vi "CAL_FLOW_SENSOR 2016.vi"(7 "Array in":refnum<k24>[](array[refnum]), 8 "error in (no error)":errorcluster, 9 "Descriptions":string[](array[string]), 11 "flow_slope_IN":dbl=51.35 format="%.2f") -> (0 "error out":errorcluster, 2 "Sensor Cluster":T1, 3 "flow_slope\nmL/min":dbl=51.35 format="%.2f", 5 "Array out":refnum<k24>[](array[refnum]))   [LabVIEW 2016]
uses:
  C:/Program Files (x86)/National Instruments/LabVIEW 2016/vi.lib/ULx/ULx_LV.dll
  Program Files (x86)/National Instruments/LabVIEW 2016/vi.lib/ULx/ULx_LV.dll
  controls/MCC DAQ Readings.ctl
  Kpro Globals.vi
  Global_SIM_switch.vi
panel:
  out "Global Flow\n Slope Valid":bool
  in  "Flow Slope":dbl format="%#_13g"
  out "Flow":dbl format="%.2f"
  in  "stop":bool
  in  "start":bool
  # "FLOW SENSOR CALIBRATION"
  # "Start Kpro flow. Allow the flow to equilibrate."
  # "After flow has equilibrated,  Press Start, simultaneously move Kpro effluent into graduated cylinder."
  # "Press Stop when 100 mL of water has been collected."
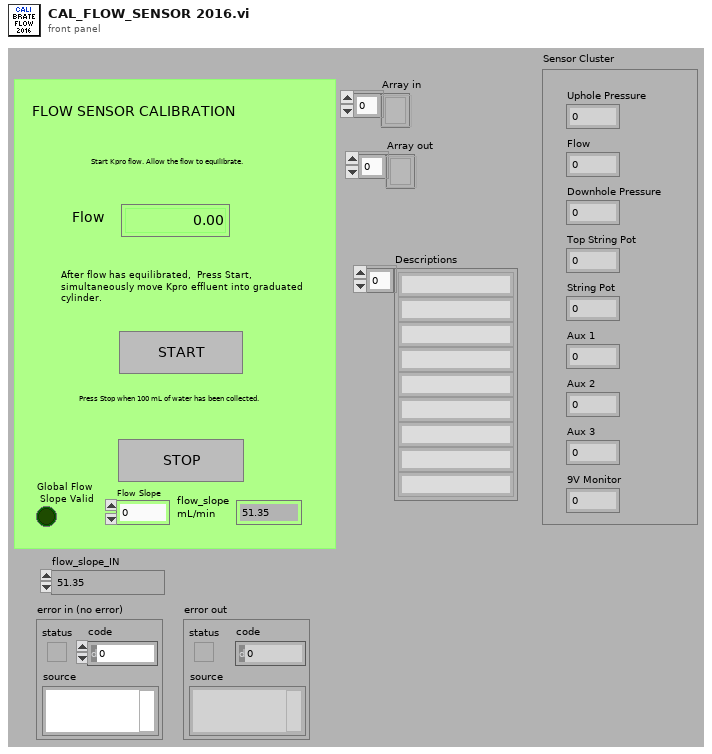
[diagram p1: front panel]
types:
  T1 = typedef "MCC DAQ Readings.ctl" = cluster{"Uphole Pressure":dbl, "Flow":dbl, "Downhole Pressure":dbl, "Top String Pot":dbl, "String Pot":dbl, "Aux 1":dbl, "Aux 2":dbl, "Aux 3":dbl, "9V Monitor":dbl}
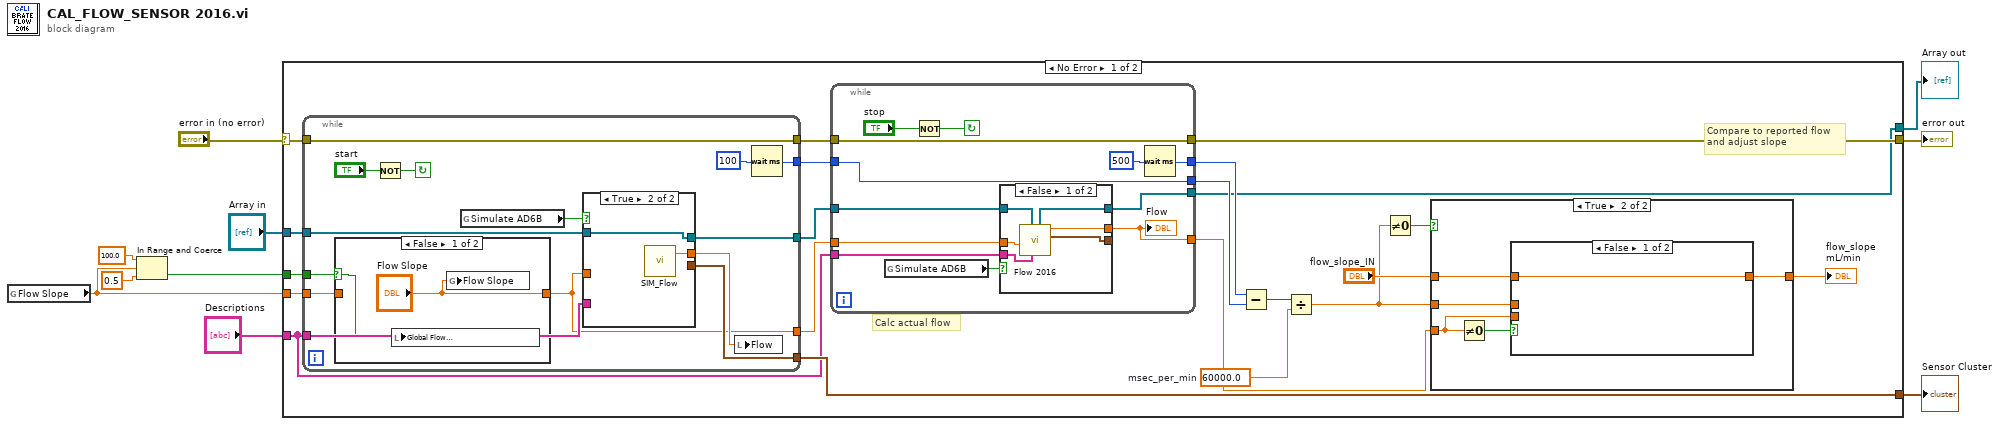
[diagram p0: block diagram]
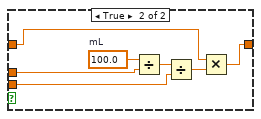
[diagram p3: hidden frame]
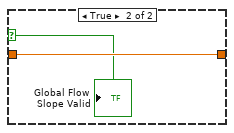
[diagram p4: hidden frame]
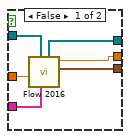
[diagram p5: hidden frame]
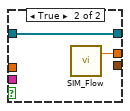
[diagram p6: hidden frame]
diagram:
  n1 = global read "Kpro Globals.vi" "Flow Slope"() -> (w2:dbl)
  n2 = In Range and Coerce(upper limit=100.0, x=w2, lower limit=0.5) -> (In Range?=w1:bool)  [unwired: 1 out]
  n3 = case shown="No Error" "error in (no error)" {
    selector: "error in (no error)" -> [w31 w93]
    tunnel: [w29 w93] -> w10
    tunnel: "Descriptions" -> [w18 _]
    tunnel: "Array in" -> [w20 w92]
    tunnel: [w19 _] -> w6
    tunnel: [w16 w92] -> w5
    tunnel: w2 -> [w12 _]
    tunnel: w1 -> [w11 _]
    frame No Error {
      w25 = 60000.0  # msec_per_min
      # "Compare to reported flow\nand adjust slope"
      # "Calc actual flow"
      n4 = while {
        tunnel: [w55] -> w30
        tunnel: w31 -> [w55]
        tunnel: [w56] -> w28
        tunnel: w18 -> [w52]
        tunnel: w20 -> [w51]
        tunnel: [w50] -> w19
        tunnel: [w49] -> w17
        tunnel: [w47] -> w15
        tunnel: w12 -> [w48]
        tunnel: w11 -> [w46]
        stop <- w58 continue-if-true
        n5 = case shown="False" w46 {
          selector: w46 -> [w60 w62]
          tunnel: w48 -> [_ w63]
          tunnel: ["Flow Slope" w63] -> w47
          frame False {
            n6 = local write "Global Flow\n Slope Valid"(w60) -> ()
            n7 = global write "Kpro Globals.vi" "Flow Slope"("Flow Slope") -> ()
          }
          frame True {
            "Global Flow\n Slope Valid" <- w62
          }
        }
        n8 = Not(x="start") -> (.not. x?=w58:bool)
        n9 = global read "Global_SIM_switch.vi" "Simulate AD6B"() -> (w54:bool)
        n10 = case shown="True" w54 {
          tunnel: [w66 w71] -> w53
          tunnel: w52 -> [w69 _]
          tunnel: w51 -> [w68 w70]
          tunnel: [w67 _] -> w50
          tunnel: w47 -> [w65 _]
          tunnel: [w64 w70] -> w49
          frame False {
            n11 = call "Flow 2016.vi"("Descriptions"=w69, "Array in"=w68, "Flow Slope"=w65) -> ("Sensor Cluster"=w67:T1, "Flow (ml/min)"=w66:dbl, "Array out"=w64:refnum<k24>[])  [unwired: 5 in]
          }
          frame True {
            n12 = call "SIM_Flow.vi"() -> ("Flow (ml/min)"=w71:dbl)  [unwired: 3 in]
          }
        }
        n13 = local write "Flow"(w53) -> ()
        n14 = Wait (ms)(milliseconds to wait=u32 100) -> (millisecond timer value=w56:u32)
      }
      n15 = while {
        tunnel: [w73] -> w21
        tunnel: w28 -> [w78]
        tunnel: [w78] -> w26
        tunnel: w30 -> [w79]
        tunnel: [w79] -> w29
        tunnel: [w81] -> w27
        tunnel: w18 -> [w76]
        tunnel: w17 -> [w75]
        tunnel: [w74] -> w16
        tunnel: w15 -> [w72]
        stop <- w83 continue-if-true
        n16 = global read "Global_SIM_switch.vi" "Simulate AD6B"() -> (w77:bool)
        n17 = Not(x="stop") -> (.not. x?=w83:bool)
        n18 = case shown="False" w77 {
          tunnel: [w86 w91] -> w73
          tunnel: w76 -> [w89 _]
          tunnel: w75 -> [w88 w90]
          tunnel: [w87 _] -> _
          tunnel: w72 -> [w85 _]
          tunnel: [w84 w90] -> w74
          frame False {
            n19 = call "Flow 2016.vi"("Descriptions"=w89, "Array in"=w88, "Flow Slope"=w85) -> ("Sensor Cluster"=w87:T1, "Flow (ml/min)"=w86:dbl, "Array out"=w84:refnum<k24>[])  [unwired: 5 in]
          }
          frame True {
            n20 = call "SIM_Flow.vi"() -> ("Flow (ml/min)"=w91:dbl)  [unwired: 3 in]
          }
        }
        "Flow" <- w73
        n21 = Wait (ms)(milliseconds to wait=u32 500) -> (millisecond timer value=w81:u32)
      }
      n22 = Subtract(x=w27, y=w26) -> (x-y=w24:u32)
      n23 = Divide(x=w24, y=w25) -> (x/y=w13:dbl)
      n24 = Not Equal To 0?(x=w13) -> (x != 0?=w14:bool)
      n25 = case shown="True" w14 {
        tunnel: w13 -> [_ w37]
        tunnel: "flow_slope_IN" -> [w32 w36]
        tunnel: [w32 w35] -> w22
        tunnel: w21 -> [_ w34]
        frame False {
        }
        frame True {
          n26 = Not Equal To 0?(x=w34) -> (x != 0?=w33:bool)
          n27 = case shown="False" w33 {
            tunnel: w37 -> [_ w44]
            tunnel: w36 -> [w38 w42]
            tunnel: [w38 w41] -> w35
            tunnel: w34 -> [_ w39]
            frame False {
            }
            frame True {
              w45 = 100.0  # mL
              n28 = Divide(x=w45, y=w44) -> (x/y=w40:dbl)
              n29 = Divide(x=w40, y=w39) -> (x/y=w43:dbl)
              n30 = Multiply(x=w42, y=w43) -> (x*y=w41:dbl)
            }
          }
        }
      }
      "flow_slope\nmL/min" <- w22
    }
    frame Error {
    }
  }
  "error out" <- w10
  "Sensor Cluster" <- w6
  "Array out" <- w5
